vi "Read TCS parameters.vi"(8 "error in (no error)":errorcluster, 11 "Telemetry in":refnum<class "Telemetry.lvclass">) -> (0 "error out":errorcluster, 2 "TCS parameters":T1, 3 "Telemetry out":refnum<class "Telemetry.lvclass">)   [LabVIEW 2018, in "Telemetry.lvclass"]
uses:
  Telemetry.lvclass
  Telemetry.lvclass/Telemetry.ctl
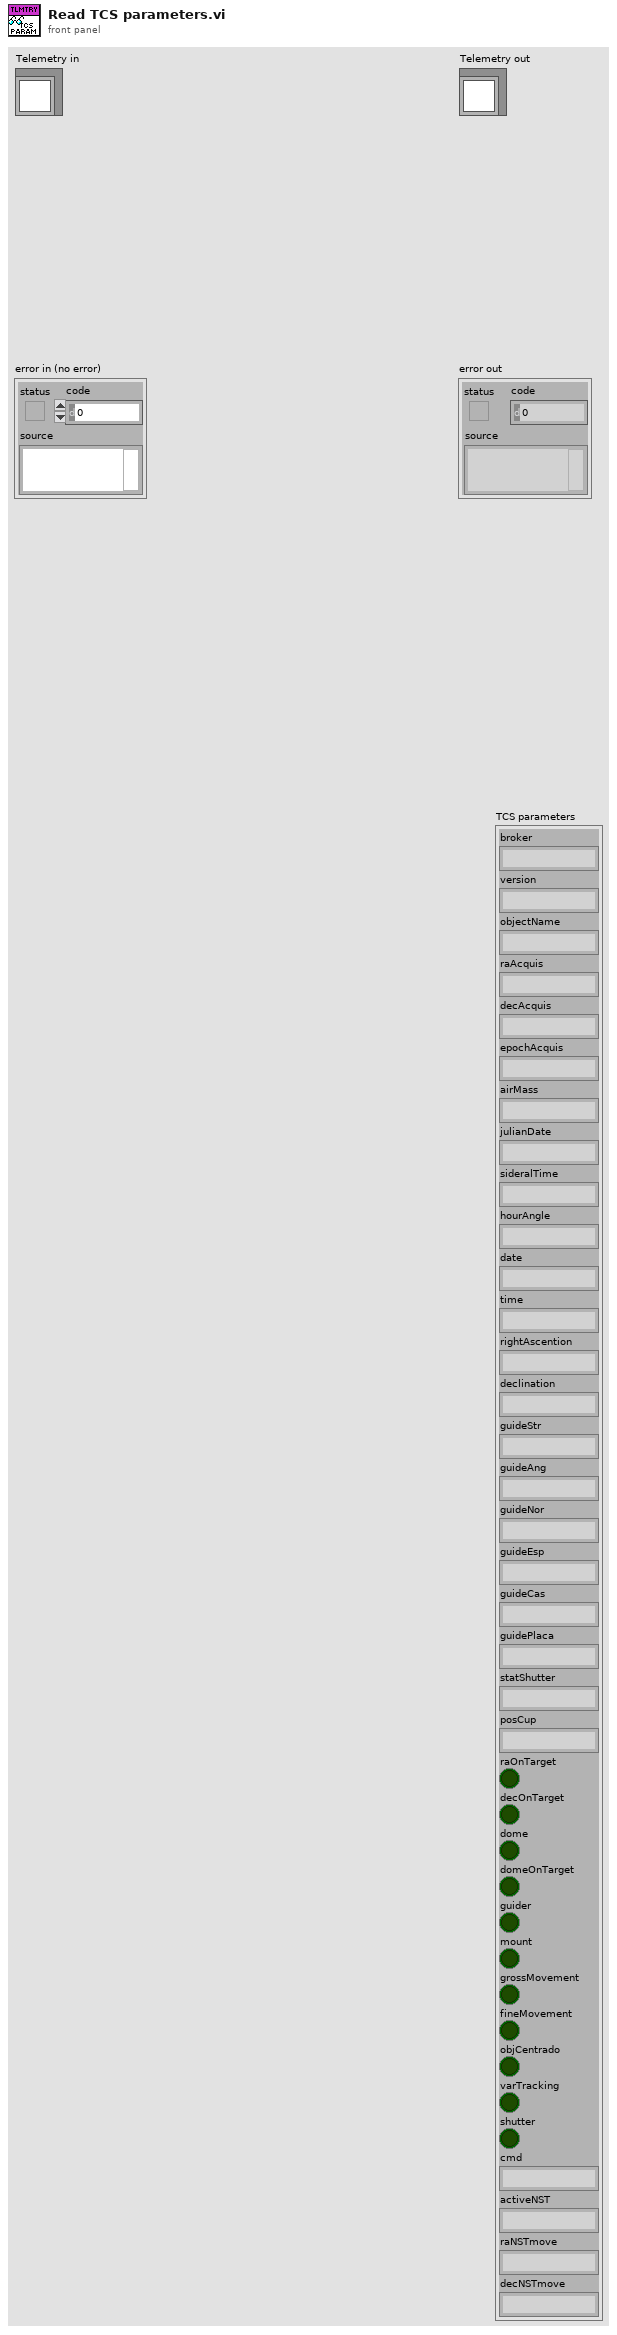
[diagram p1: front panel]
types:
  T1 = cluster{"broker":string, "version":string, "objectName":string, "raAcquis":string, "decAcquis":string, "epochAcquis":string, "airMass":string, "julianDate":string, "sideralTime":string, "hourAngle":string, "date":string, "time":string, "rightAscention":string, "declination":string, "guideStr":string, "guideAng":string, "guideNor":string, "guideEsp":string, "guideCas":string, "guidePlaca":string, "statShutter":string, "posCup":string, "raOnTarget":bool, "decOnTarget":bool, "dome":bool, "domeOnTarget":bool, "guider":bool, "mount":bool, "grossMovement":bool, "fineMovement":bool, "objCentrado":bool, "varTracking":bool, "shutter":bool, "cmd":string, "activeNST":string, "raNSTmove":string, "decNSTmove":string}
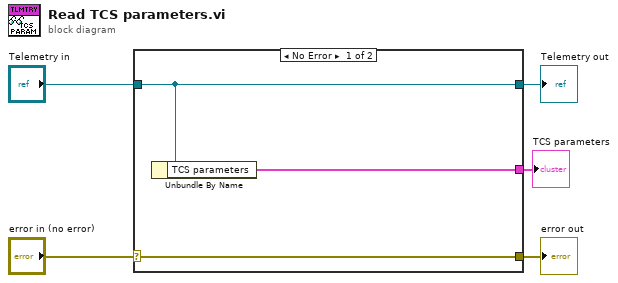
[diagram p0: block diagram]
diagram:
  n1 = case shown="No Error" "error in (no error)" {
    selector: "error in (no error)" -> [w8 w9]
    tunnel: [w8 w9] -> w4
    tunnel: [w7 w10] -> w2
    tunnel: "Telemetry in" -> [w7 w10]
    tunnel: [w6 _] -> w1
    frame No Error {
      n2 = Unbundle By Name(w7) -> ("TCS parameters"=w6:T1)
    }
    frame Error {
    }
  }
  "error out" <- w4
  "Telemetry out" <- w2
  "TCS parameters" <- w1
